vi "Main.vi"() -> ()   [LabVIEW 2017]
doc: "The myRIO Project template acquires acceleration data from the onboard accelerometer and displays the changes of acceleration values in a waveform chart."
uses:
  <vilib>/myRIO/Common/Instrument Driver Framework/myRIO v1.0/Encoder/typedefs/Encoder Count Direction Enum.ctl
  <vilib>/myRIO/Instrument Drivers/Onboard IO/PWM/typedefs/PWM Reference.ctl
  <vilib>/myRIO/Common/Instrument Driver Framework/Utilities/typedefs/myRIO Generic Hardware Reference.ctl
  <vilib>/myRIO/Common/Instrument Driver Framework/Utilities/typedefs/Hardware Version Enum.ctl
  <vilib>/myRIO/Common/Instrument Driver Framework/Utilities/typedefs/myRIO v1.0 Reference.ctl
  <vilib>/myRIO/Common/Instrument Driver Framework/Utilities/typedefs/Generic FPGA Reference.ctl
  <vilib>/myRIO/Common/Instrument Driver Framework/myRIO v1.0/PWM/typedefs/PWM Channels Enum.ctl
  <vilib>/myRIO/Instrument Drivers/Onboard IO/PWM/typedefs/PWM Configuration.ctl
  <vilib>/userdefined/High Color/nirio_resource_hc.ctl
  <vilib>/myRIO/Common/Instrument Driver Framework/Utilities/vis/Is FPGA Ref Available.vi
  <vilib>/myRIO/Common/Instrument Driver Framework/myRIO v1.0/PWM/vis/myRIO v1.1 Open PWM.vi
  <vilib>/myRIO/Instrument Drivers/Onboard IO/PWM/vis/Set Duty Cycle and Frequency.vi
  <vilib>/myRIO/Common/Instrument Driver Framework/Utilities/vis/Validate Channels.vi
  <vilib>/myRIO/Common/Instrument Driver Framework/myRIO v1.0/PWM/vis/myRIO v1.0 Reserve PWM.vi
  <vilib>/myRIO/Common/Instrument Driver Framework/myRIO v1.0/UART/vis/myRIO v1.0 Close UART.vi
  <vilib>/myRIO/Common/Instrument Driver Framework/myRIO v1.0/PWM/vis/myRIO v1.0 Build MUX Configuration PWM.vi
  <vilib>/myRIO/Common/Instrument Driver Framework/myRIO v1.0/Resource Manager/vis/myRIO v1.0 Reserve Channel List.vi
  <vilib>/myRIO/Common/Instrument Driver Framework/myRIO v1.0/Resource Manager/vis/myRIO v1.0 Create Configuration List.vi
  <vilib>/myRIO/Common/Instrument Driver Framework/myRIO v1.0/Resource Manager/vis/myRIO v1.0 Reserve Channel.vi
  <vilib>/myRIO/Common/Instrument Driver Framework/myRIO v1.0/Resource Manager/vis/myRIO v1.0 Unreserve Channel.vi
  <vilib>/myRIO/Common/Instrument Driver Framework/myRIO v1.0/Resource Manager/vis/myRIO v1.0 Build Mutex Name.vi
  <vilib>/Utility/VariantDataType/GetNumericInfo.vi
  <vilib>/Utility/error.llb/Error Cluster From Error Code.vi
  <vilib>/myRIO/Common/Instrument Driver Framework/myRIO v1.0/myRIO v1.1 Open.vi
  <vilib>/myRIO/Common/Instrument Driver Framework/Utilities/vis/IO Manager.vi
  <vilib>/myRIO/Common/Instrument Driver Framework/Utilities/vis/Configuration Manager.vi
  <vilib>/myRIO/Common/Instrument Driver Framework/myRIO v1.0/Resource Manager/vis/myRIO v1.0 Configure IO.vi
  <vilib>/myRIO/Common/Instrument Driver Framework/myRIO v1.0/myRIO v1.0 Close.vi
  <vilib>/myRIO/Common/Instrument Driver Framework/myRIO v1.0/PWM/vis/myRIO v1.0 Write PWM.vi
  <vilib>/myRIO/Common/Instrument Driver Framework/Utilities/vis/FPGA Ref Manager.vi
  <vilib>/myRIO/Common/Instrument Driver Framework/myRIO v1.0/myRIO v1.0 Reset FPGA.vi
  <vilib>/myRIO/Common/Instrument Driver Framework/myRIO v1.0/IRQ/vis/myRIO v1.0 IRQ Info FGV.vi
  <vilib>/myRIO/Common/Instrument Driver Framework/myRIO v1.0/IRQ/vis/myRIO v1.0 Timer IRQ Info FGV.vi
  <vilib>/myRIO/Common/Instrument Driver Framework/myRIO v1.0/IRQ/vis/myRIO v1.0 ISR Agent.vi
  <vilib>/myRIO/Express VI/Onboard IO/PWM/PWM Express VI.xnode
  <vilib>/myRIO/Instrument Drivers/Onboard IO/PWM/vis/myRIO PWM Open.xnode
  <vilib>/myRIO/Instrument Drivers/Utilities/Utilities.lvlib
  <vilib>/myRIO/Instrument Drivers/Onboard IO/PWM/PWM.lvlib
panel:
  out "Output String":string
  out "Encoder Output":T2
  out "Loop Iteration":i32
  in  "X Axis":T3
  in  "Y Axis":cluster{"Frequency":dbl, "FWD/RVS":bool}
  in  "stop":bool
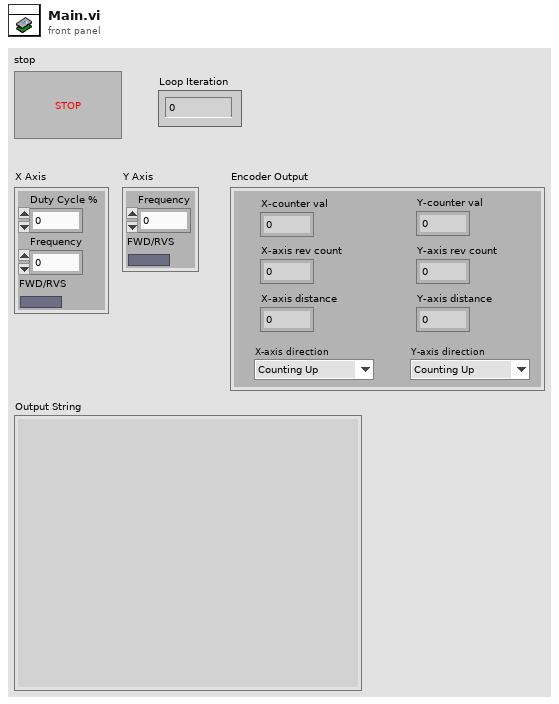
[diagram p1: front panel]
types:
  T1 = typedef "Encoder Count Direction Enum.ctl" = enum16{"Counting Up", "Counting Down"}
  T2 = cluster{"Y-axis rev count":dbl, "Y-axis distance":dbl, "X-axis rev count":dbl, "X-axis distance":dbl, "Y-axis direction":T1, "X-axis direction":T1, "X-counter val":i32, "Y-counter val":i32}
  T3 = cluster{"Duty Cycle % ":dbl, "Frequency":dbl, "FWD/RVS":bool}
  T4 = cluster{dbl, "X-axis distance":dbl, "Duty Cycle % ":dbl, "Frequency":dbl, "Y-axis distance":dbl, "Frequency":dbl}
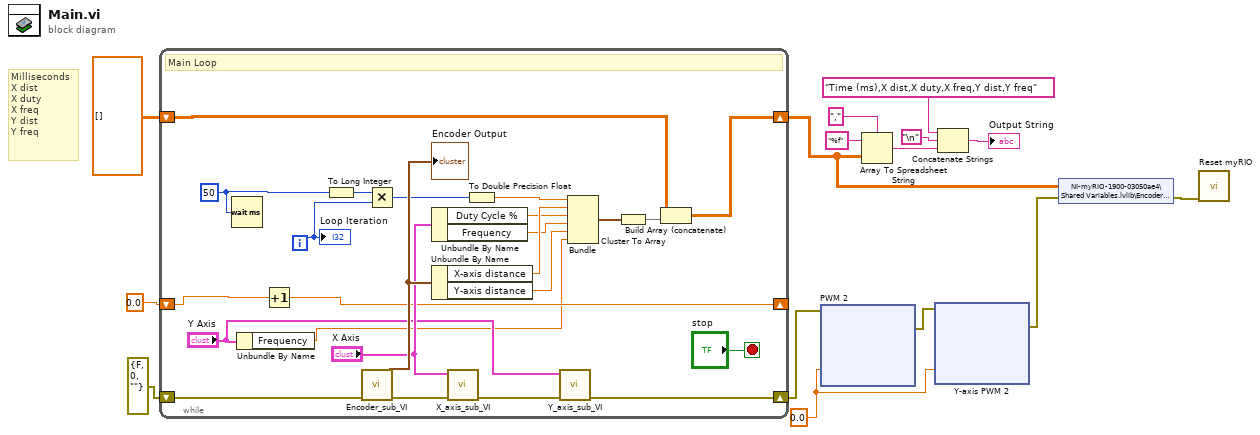
[diagram p0: block diagram]
diagram:
  w1 = 0.0 ("Frequency [Hz]")
  # "Milliseconds\nX dist\nX duty\nX freq\nY dist\nY freq"
  n1 = while {
    shift-right: [w38] -> w15
    shift-left: errorcluster {"status"=FALSE, "code"=0, "source"=""} ("error in (no error)") -> [w39]
    shift-right: [w20] -> w4
    shift-left: dbl[][] [] -> [w22]
    shift-right: [w18] -> _
    shift-left: 0.0 -> [w21]
    i -> [w19]
    stop <- "stop" stop-if-true
    w33 = u32 50 ("milliseconds to wait")
    # "Main Loop"
    n2 = Wait (ms)(milliseconds to wait=w33) -> ()  [unwired: 1 out]
    n3 = Unbundle By Name("Y Axis") -> ("Frequency"=w16:dbl)
    n4 = Increment(x=w21) -> (x+1=w18:dbl)
    n5 = To Long Integer(number=w33) -> (32bit integer=w32:i32)
    n6 = call "Encoder_sub_VI.vi"("error in (no error)"=w39) -> ("error out"=w35:errorcluster, "Encoder Output"=w34:T2)  [unwired: 9 in]
    "Encoder Output" <- w34
    n7 = Multiply(x=w32, y=w19) -> (x*y=w30:i32)
    n8 = Unbundle By Name("X Axis") -> ("Duty Cycle %"=w24:dbl, "Frequency"=w23:dbl)
    n9 = Unbundle By Name(w34) -> ("X-axis distance"=w28:dbl, "Y-axis distance"=w26:dbl)
    n10 = call "X_axis_sub_VI.vi"("error in (no error)"=w35, "X Axis"="X Axis") -> ("error out"=w36:errorcluster)  [unwired: 9 in]
    n11 = To Double Precision Float(number=w30) -> (double precision float=w29:dbl)
    n12 = call "Y_axis_sub_VI.vi"("error in (no error)"=w36, "Y Axis"="Y Axis") -> ("error out"=w38:errorcluster)  [unwired: 9 in]
    n13 = Bundle(w29, "X-axis distance"=w28, "Duty Cycle %"=w24, "Frequency"=w23, "Y-axis distance"=w26, "Frequency"=w16) -> (w31:T4)  [unwired: 1 in]
    n14 = Cluster To Array(cluster=w31) -> (array=w27:dbl[])
    n15 = Build Array (concatenate)(w22, w27) -> (w20:dbl[][])
    "Loop Iteration" <- w19
  }
  n16 = xnode "PWM 2"("Frequency [Hz]"=w1, "error in (no error)"=w15) -> ("error out"=w3:errorcluster)
  n17 = Array To Spreadsheet String(delimiter (Tab)=",", array=w4, 3:"%f" ("format string")) -> (spreadsheet string=w12:string)
  n18 = xnode "Y-axis PWM 2"("Frequency [Hz]"=w1, "error in (no error)"=w3) -> ("error out"=w2:errorcluster)
  n19 = Concatenate Strings("Time (ms),X dist,X duty,X freq,Y dist,Y freq", "\n", w12) -> (→"Output String":string)
  n20 = shared-variable "NI-myRIO-1900-03050ae4\\Shared Variables.lvlib\\Encoder Data"(w4, error in=w2) -> (error out=w5:errorcluster)
  n21 = call <vilib>:"Reset myRIO.vi"("error in (no error)"=w5) -> ()  [unwired: 10 in, 1 out]
